vi "SDG60UploadArbWaveform2.vi"(0 "VISA resource name":refnum<visa-resource-name>="USB0::0xF4EC::0x1101::SDG6XEBC5R0119::INSTR", 1 "WFM Length (20E6)":i32=20000000, 2 "Readback":bool, 3 "WFM (Column) Number":i32, 5 "WFM Numer ARBn":u32=1, 9 "Timeout (40000 ms)":u32=40000, 11 "error in (no error)":errorcluster, 12 "Array WFM":i16[](array[numeric])=[1000, 2000, 3000, 4000, 5000, 6000, 7000, 8000], 13 "Number of retries":i32=1, 14 "WFM Source":u16(ring) items=["Single file", "Split files", "Array"]) -> (4 "VISA resource name out":refnum<visa-resource-name>, 6 "Readback error":bool, 10 "Total time":dbl format="%#_15g", 15 "error out":errorcluster)   [LabVIEW 2018]
doc: "Creates and saves an arbitrary (user-defined) waveform in non-volatile memory, then selects it for output."
uses:
  <vilib>/Utility/file.llb/Read From Spreadsheet File (I64).vi
panel:
  out "Rdbk WFM str":string
  out "WFM str":string
  out "WFM to arr time":dbl format="%#_15g"
  out "Arr to str time":dbl format="%#_15g"
  out "Upload time":dbl format="%#_15g"
  out "Attempts (0: First)":i32
  in  "WFM Path":path=path "C:/Data/_SoftDevelopment/SDG6000/WFMTst20E6PtsInt.txt"
  # "The input range for ARB data is: -32767..+32767 (must be integers)\n\nC1 hardcoded within vi as needs to have a channel assigned to be uploaded. \nCan then be selected for either channel.\n\nUpon overwrite of name with new WFM, still needs to be selected\notherwise will still use old WFM with that name. If WFM has been selected, and then gets deleted off \nC drive, will still output WFM on that channel\n\nTesting uploads of large WFMS.\n8M: All ok, can have 2 separate WFMs on 2 channels and upload more\n16M: Can have 2 separate WFMs on 2 channels, storage space limits 3rd upload\n          of 16M points, but can upload 8M and switch fine between them all.\n20M: Can have 20M on both channels, but then no storage space to upload third\n\nVi will write the file with a small (16B bin file on device) file (overwriting any WFM \n           previously with that name),  then write the WFM selected with the one chosen to \n           upload.  This means you don't need to clear space off the device, as long as the \n           name of the WFM is already on the device. If a new name is chosen, then will have to manually delete the old WFM, \n           or use SDG60DeleteAllWaveforms vi, if need to free up space.\n\nIf too large a waveform is uploaded (over 20M), generator will crash requiring manual power\ncycle\n\nIf storage full, will beep on generator and say storage full, but not give any error through \nlabview. Waveform won't ovewrite others when uploading if storage full.\n\nSingle pixel test, (oscilloscope limited to 200MHz) , for 20M points. the single pixel did go to\n +32767, Pk-Pk on scope was 3.36V when should be 4.0 Vpp. The burst width (FWHM) was \n3.962 ns. RMS was 1.99 V. 3.2ns FWHM on 2GHz infiinium scope (no longer limited by scope)"
  # "Max: 20E6 (decimal)"
  # "Rdbk fails if WFM length>30000, because str read via VISA is incomplete\nand crashes USB. requiring powercycle\ngenerator. Needs further investigation"
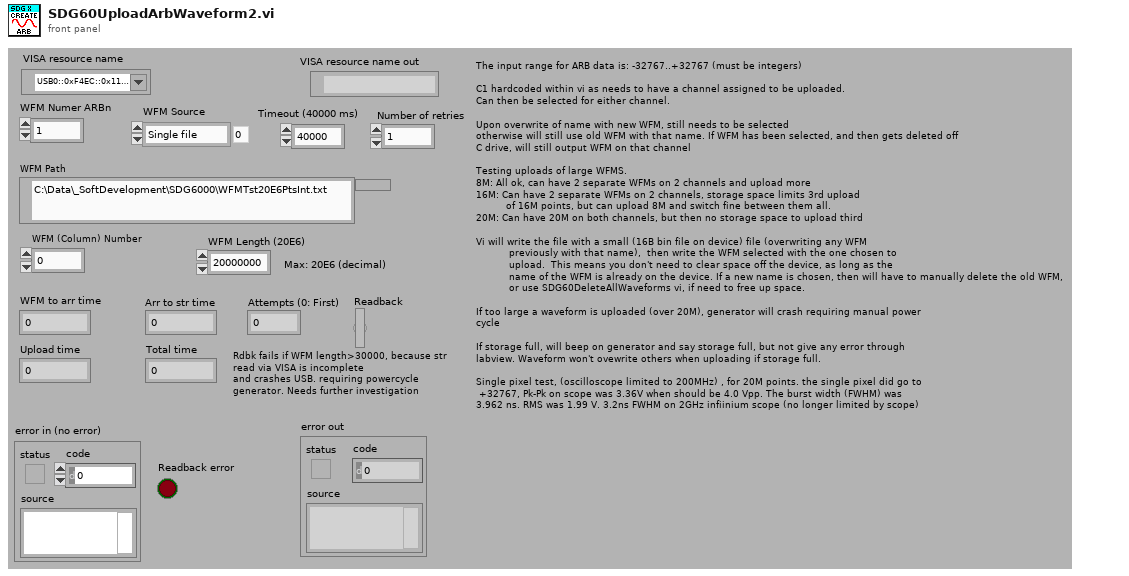
[diagram p1: front panel]
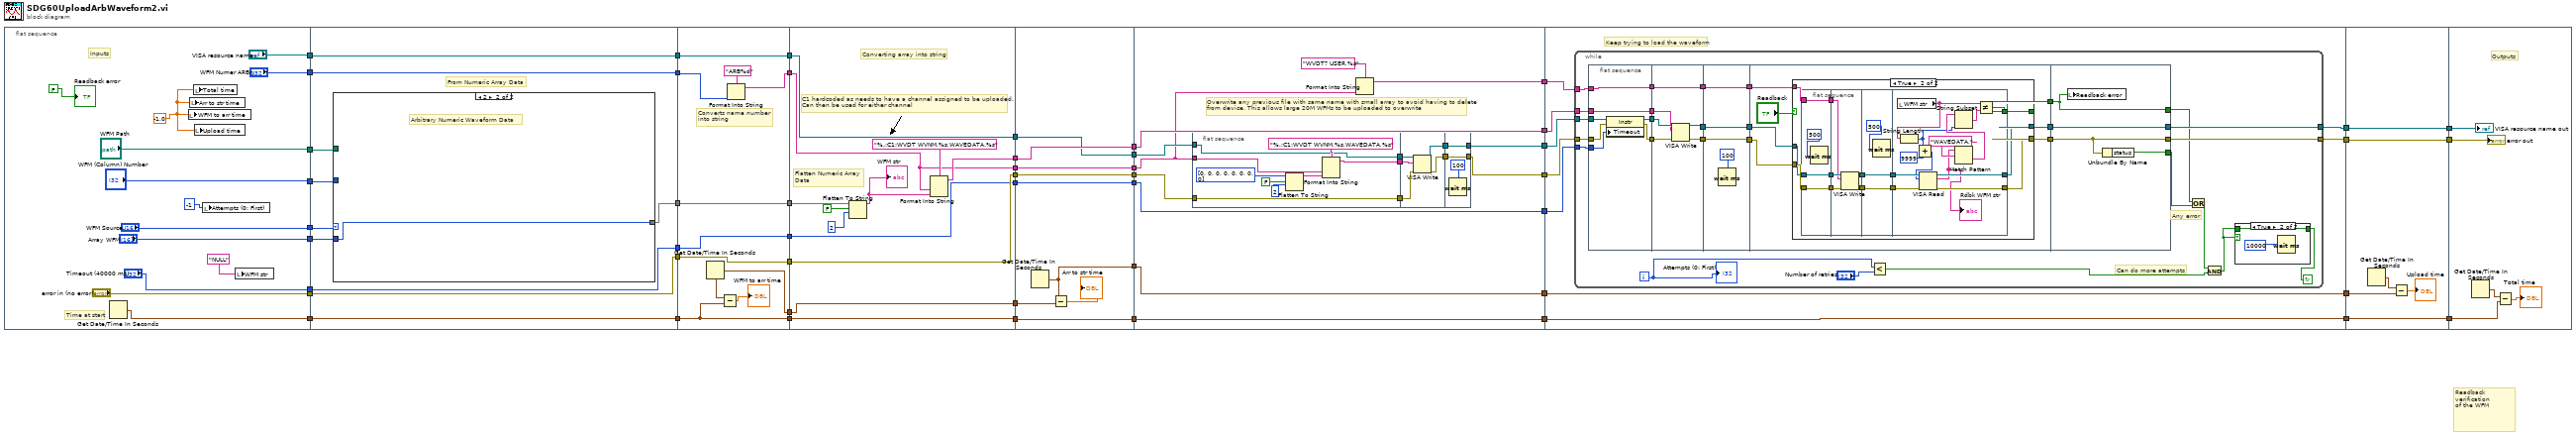
[diagram p0: block diagram]
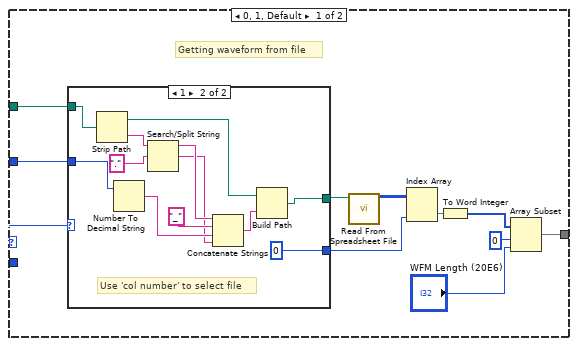
[diagram p2: hidden frame]
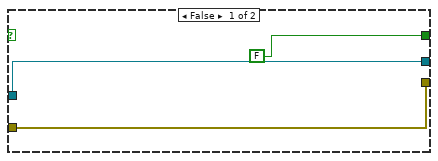
[diagram p5: hidden frame]
diagram:
  # "Readback verification\nof the WFM"
  n1 = flat-sequence {
    tunnel: ["WFM Source"] -> w10
    tunnel: ["Array WFM"] -> w9
    tunnel: ["WFM Path"] -> w8
    tunnel: ["WFM (Column) Number"] -> w7
    tunnel: ["VISA resource name"] -> w6
    tunnel: ["error in (no error)"] -> w4
    tunnel: ["Timeout (40000 ms)"] -> w3
    tunnel: [w56] -> w2
    tunnel: ["WFM Numer ARBn"] -> w5
    tunnel: w10 -> [w73]
    tunnel: w9 -> [w72]
    tunnel: [w71] -> w50
    tunnel: w8 -> [w70]
    tunnel: w7 -> [w69]
    tunnel: [w68] -> w48
    tunnel: w6 -> [w68]
    tunnel: [w67] -> w46
    tunnel: w5 -> [w67]
    tunnel: [w66] -> w44
    tunnel: w4 -> [w66]
    tunnel: [w65] -> w42
    tunnel: w3 -> [w65]
    tunnel: [w64] -> w40
    tunnel: w2 -> [w64]
    tunnel: w50 -> [w109]
    tunnel: [w109] -> w49
    tunnel: w48 -> [w108]
    tunnel: [w108] -> w47
    tunnel: w46 -> [w100]
    tunnel: [w101] -> w45
    tunnel: w44 -> [w104]
    tunnel: [w104] -> w43
    tunnel: w42 -> [w105]
    tunnel: [w105] -> w41
    tunnel: w40 -> [w106]
    tunnel: [w106] -> w39
    tunnel: [w103] -> w25
    tunnel: w49 -> [w113]
    tunnel: [w115] -> w38
    tunnel: [w120] -> w37
    tunnel: [w119] -> w36
    tunnel: [w118] -> w35
    tunnel: w47 -> [w120]
    tunnel: w45 -> [w110]
    tunnel: w43 -> [w119]
    tunnel: w41 -> [w118]
    tunnel: w39 -> [w117]
    tunnel: [w117] -> w34
    tunnel: [w116] -> w26
    tunnel: w25 -> [w116]
    tunnel: [w110] -> w11
    tunnel: w38 -> [w130]
    tunnel: [w130] -> w24
    tunnel: w37 -> [w129]
    tunnel: [w129] -> w22
    tunnel: w36 -> [w128]
    tunnel: [w128] -> w20
    tunnel: w35 -> [w127]
    tunnel: [w127] -> w18
    tunnel: w34 -> [w123]
    tunnel: [w123] -> w16
    tunnel: [w125] -> w14
    tunnel: w26 -> [w124]
    tunnel: [w122] -> w12
    tunnel: w11 -> [w122]
    tunnel: w24 -> [w146]
    tunnel: [w146] -> w23
    tunnel: w22 -> [w135]
    tunnel: [w134] -> w21
    tunnel: w20 -> [w139]
    tunnel: [w138] -> w19
    tunnel: w18 -> [w145]
    tunnel: [w145] -> w17
    tunnel: w16 -> [w144]
    tunnel: [w144] -> w15
    tunnel: w14 -> [w143]
    tunnel: [w143] -> w13
    tunnel: w12 -> [w132]
    tunnel: [w131] -> w1
    tunnel: [w165] -> w33
    tunnel: [w166] -> w31
    tunnel: w23 -> [w172]
    tunnel: w21 -> [w171]
    tunnel: w19 -> [w170]
    tunnel: w17 -> [w169]
    tunnel: w15 -> [w168]
    tunnel: [w168] -> w29
    tunnel: w13 -> [w167]
    tunnel: [w167] -> w27
    tunnel: w1 -> [w164]
    tunnel: w33 -> [w278]
    tunnel: [w278] -> w32
    tunnel: w31 -> [w277]
    tunnel: [w277] -> w30
    tunnel: w29 -> [w275]
    tunnel: [w275] -> w28
    tunnel: w27 -> [w274]
    tunnel: w32 -> [w283]
    tunnel: w30 -> [w282]
    tunnel: w28 -> [w279]
    frame #0 {
      w55 = -1.0
      # "Inputs"
      # "Time at start"
      n2 = Get Date/Time In Seconds() -> (seconds since 1Jan1904=w56:timestamp)
      n3 = local write "WFM to arr time"(w55) -> ()
      n4 = local write "Arr to str time"(w55) -> ()
      n5 = local write "Total time"(w55) -> ()
      n6 = local write "Upload time"(w55) -> ()
      n7 = local write "Attempts (0: First)"(-1) -> ()
      n8 = local write "WFM str"("NULL") -> ()
      "Readback error" <- FALSE
    }
    frame #1 {
      # "From Numeric Array Data"
      n9 = case shown="2" w73 {
        selector: w73 -> [w82 _]
        tunnel: [w77 w99] -> w71
        tunnel: w72 -> [_ w99]
        tunnel: w70 -> [w76 _]
        tunnel: w69 -> [w75 _]
        frame 0, 1, Default {
          # "Getting waveform from file"
          n10 = case shown="1" w82 {
            tunnel: w76 -> [w86 w98]
            tunnel: w75 -> [w85 w95]
            tunnel: [w86 w88] -> w80
            tunnel: [w85 0 ("x")] -> w79
            frame 0, Default {
              # "File contains multiple wfms"
            }
            frame 1 {
              # "Use 'col number' to select file"
              n11 = Strip Path(path=w98) -> (stripped path=w90:path, name=w96:string)
              n12 = Number To Decimal String(number=w95) -> (decimal integer string=w92:string)  [unwired: 1 in]
              n13 = Search/Split String(string=w96, search string/char (-)=".") -> (substring before match=w94:string, match + rest of string=w91:string)  [unwired: 1 in, 1 out]
              n14 = Concatenate Strings(w94, "_", w92, w91) -> (w89:string)
              n15 = Build Path(base path=w90, name or relative path=w89) -> (appended path=w88:path)
            }
          }
          n16 = call-poly <vilib>:"Read From Spreadsheet File.vi"("file path (dialog if empty)"=w80) -> ("all rows"=w81:i64[][])  [unwired: 6 in, 4 out]
          n17 = Index Array(array=w81, index (col)=w79) -> (element=w78:i64[])  [unwired: 1 in]
          n18 = To Word Integer(number=w78) -> (16bit integer=w84:i16[])
          n19 = Array Subset(array=w84, index=0 ("x"), length="WFM Length (20E6)") -> (w77:i16[])
        }
        frame 2 {
          # "Arbitrary Numeric Waveform Data"
        }
      }
    }
    frame #2 {
      # "Converts name number \ninto string"
      n20 = Get Date/Time In Seconds() -> (seconds since 1Jan1904=w103:timestamp)
      n21 = Subtract(x=w103, y=w106) -> (x-y=→"WFM to arr time":dbl)
      n22 = Format Into String(format string="ARB%d", w100) -> (resulting string=w101:string)  [unwired: 2 in, 1 out]
    }
    frame #3 {
      # "Converting array into string"
      # "C1 hardcoded as needs to have a channel assigned to be uploaded. \nCan then be used for either channel"
      # "Flatten Numeric Array \nData"
      n23 = Flatten To String(anything=w113, prepend array or string size? (T)=FALSE, byte order (0:big-endian, network order)=2) -> (data string=w111:string)  [unwired: 1 in, 2 out]
      "WFM str" <- w111
      n24 = Format Into String(format string="%.;C1:WVDT WVNM,%s,WAVEDATA,%s", w110, w111) -> (resulting string=w115:string)  [unwired: 2 in, 1 out]
    }
    frame #4 {
      n25 = Get Date/Time In Seconds() -> (seconds since 1Jan1904=w125:timestamp)
      n26 = Subtract(x=w125, y=w124) -> (x-y=→"Arr to str time":dbl)
    }
    frame #5 {
      # "Overwrite any previous file with same name with small array to avoid having to delete\nfrom device. This allows large 20M WFMs to be uploaded to overwrite"
      n27 = flat-sequence {
        tunnel: w132 -> [w154]
        tunnel: [w149] -> w142
        tunnel: w139 -> [w148]
        tunnel: [w148] -> w141
        tunnel: w135 -> [w147]
        tunnel: [w147] -> w137
        tunnel: w142 -> [w160]
        tunnel: w141 -> [w159]
        tunnel: [w158] -> w140
        tunnel: w137 -> [w157]
        tunnel: [w156] -> w136
        tunnel: [w162] -> w138
        tunnel: w140 -> [w162]
        tunnel: [w161] -> w134
        tunnel: w136 -> [w161]
        frame #0 {
          n28 = Flatten To String(anything=i16[] [0, 0, 0, 0, 0, 0, 0, 0] ("Array WFM DUMMY"), prepend array or string size? (T)=FALSE, byte order (0:big-endian, network order)=2) -> (data string=w151:string)  [unwired: 1 in, 2 out]
          n29 = Format Into String(format string="%.;C1:WVDT WVNM,%s,WAVEDATA,%s", w154, w151) -> (resulting string=w149:string)  [unwired: 2 in, 1 out]
        }
        frame #1 {
          n30 = VISA Write(VISA resource name=w157, write buffer=w160, error in (no error)=w159) -> (VISA resource name out=w156:refnum<visa-resource-name>, error out=w158:errorcluster)  [unwired: 1 out]
        }
        frame #2 {
          n31 = Wait (ms)(milliseconds to wait=100 ("x")) -> ()  [unwired: 1 out]
        }
      }
      n32 = Format Into String(format string="WVDT? USER,%s", w132) -> (resulting string=w131:string)  [unwired: 2 in, 1 out]
    }
    frame #6 {
      # "Keep trying to load the waveform"
      n33 = while {
        tunnel: w172 -> [w200]
        tunnel: w171 -> [w199]
        tunnel: w170 -> [w198]
        tunnel: [w197] -> w165
        tunnel: [w196] -> w166
        tunnel: w169 -> [w188]
        tunnel: w164 -> [w187]
        i -> [w179]
        stop <- w173 continue-if-true
        # "Can do more attempts"
        # "Any error"
        n34 = flat-sequence {
          tunnel: w200 -> [w210]
          tunnel: w198 -> [w207]
          tunnel: w199 -> [w209]
          tunnel: [w208] -> w191
          tunnel: [w206] -> w190
          tunnel: [w210] -> w189
          tunnel: w188 -> [w205]
          tunnel: w187 -> [w204]
          tunnel: [w204] -> w184
          tunnel: [w212] -> w195
          tunnel: [w213] -> w194
          tunnel: w191 -> [w215]
          tunnel: w190 -> [w216]
          tunnel: w189 -> [w214]
          tunnel: [w211] -> w185
          tunnel: w184 -> [w211]
          tunnel: w195 -> [w218]
          tunnel: w194 -> [w219]
          tunnel: [w219] -> w193
          tunnel: [w218] -> w192
          tunnel: [w217] -> w186
          tunnel: w185 -> [w217]
          tunnel: w193 -> [w227]
          tunnel: w192 -> [w226]
          tunnel: w186 -> [w223]
          tunnel: [w224] -> w183
          tunnel: [w225] -> w182
          tunnel: [w221] -> w181
          tunnel: [w270] -> w176
          tunnel: [w272] -> w196
          tunnel: [w271] -> w197
          tunnel: w183 -> [w271]
          tunnel: w182 -> [w272]
          tunnel: w181 -> [w269]
          tunnel: [w269] -> w175
          frame #0 {
            n35 = property class="Instr"(reference=w209, error in=w207, "Timeout"=w205) -> (reference out=w208:refnum<visa-resource-name>, error out=w206:errorcluster)
          }
          frame #1 {
            n36 = VISA Write(VISA resource name=w215, write buffer=w214, error in (no error)=w216) -> (VISA resource name out=w213:refnum<visa-resource-name>, error out=w212:errorcluster)  [unwired: 1 out]
          }
          frame #2 {
            n37 = Wait (ms)(milliseconds to wait=100 ("x")) -> ()  [unwired: 1 out]
          }
          frame #3 {
            n38 = case shown="True" "Readback" {
              tunnel: w226 -> [w228 w237]
              tunnel: w227 -> [w229 w236]
              tunnel: [w229 w235] -> w225
              tunnel: [w228 w234] -> w224
              tunnel: [FALSE w233] -> w221
              tunnel: w223 -> [_ w232]
              frame False {
              }
              frame True {
                n39 = flat-sequence {
                  tunnel: [w246] -> w243
                  tunnel: [w245] -> w242
                  tunnel: w237 -> [w246]
                  tunnel: w236 -> [w245]
                  tunnel: w232 -> [w244]
                  tunnel: [w244] -> w231
                  tunnel: w243 -> [w251]
                  tunnel: w242 -> [w252]
                  tunnel: [w249] -> w241
                  tunnel: [w250] -> w240
                  tunnel: w231 -> [w248]
                  tunnel: w241 -> [w255]
                  tunnel: w240 -> [w254]
                  tunnel: [w255] -> w239
                  tunnel: [w254] -> w238
                  tunnel: w239 -> [w266]
                  tunnel: w238 -> [w268]
                  tunnel: [w263] -> w234
                  tunnel: [w267] -> w235
                  tunnel: [w264] -> w233
                  frame #0 {
                    n40 = Wait (ms)(milliseconds to wait=500 ("x")) -> ()  [unwired: 1 out]
                  }
                  frame #1 {
                    n41 = VISA Write(VISA resource name=w252, write buffer=w248, error in (no error)=w251) -> (VISA resource name out=w250:refnum<visa-resource-name>, error out=w249:errorcluster)  [unwired: 1 out]
                  }
                  frame #2 {
                    n42 = Wait (ms)(milliseconds to wait=500 ("x")) -> ()  [unwired: 1 out]
                  }
                  frame #3 {
                    n43 = local read "WFM str"() -> (w261:string)
                    n44 = String Length(string=w261) -> (length=w259:i32)
                    n45 = Add(x=w259, y=9999 ("x")) -> (x+y=w257:i32)
                    n46 = VISA Read(VISA resource name=w268, byte count=w257, error in (no error)=w266) -> (VISA resource name out=w267:refnum<visa-resource-name>, read buffer=w256:string, error out=w263:errorcluster)  [unwired: 1 out]
                    "Rdbk WFM str" <- w256
                    n47 = Match Pattern(string=w256, regular expression="WAVEDATA,") -> (after substring=w260:string)  [unwired: 1 in, 3 out]
                    n48 = String Subset(string=w260, length (rest)=w259) -> (substring=w258:string)  [unwired: 1 in]
                    n49 = Not Equal?(x=w261, y=w258) -> (x != y?=w264:bool)
                  }
                }
              }
            }
          }
          frame #4 {
            n50 = local write "Readback error"(w269) -> ()
            n51 = Unbundle By Name(w271) -> ("status"=w270:bool)
          }
        }
        n52 = Less?(x=w179, y="Number of retries") -> (x < y?=w178:bool)
        n53 = Or(x=w175, y=w176) -> (x .or. y?=w177:bool)
        n54 = And(x=w177, y=w178) -> (x .and. y?=w174:bool)
        n55 = case shown="True" w174 {
          tunnel: w174 -> [w201 w202]
          tunnel: [w201 w202] -> w173
          frame False {
          }
          frame True {
            n56 = Wait (ms)(milliseconds to wait=10000 ("x")) -> ()  [unwired: 1 out]
          }
        }
        "Attempts (0: First)" <- w179
      }
    }
    frame #7 {
      n57 = Get Date/Time In Seconds() -> (seconds since 1Jan1904=w276:timestamp)
      n58 = Subtract(x=w276, y=w274) -> (x-y=→"Upload time":dbl)
    }
    frame #8 {
      # "Outputs"
      n59 = Get Date/Time In Seconds() -> (seconds since 1Jan1904=w281:timestamp)
      n60 = Subtract(x=w281, y=w279) -> (x-y=→"Total time":dbl)
      "VISA resource name out" <- w282
      "error out" <- w283
    }
  }
